vi "Data Array Length.vi"(10 "Read Tank Press":bool, 11 "Read Aux Flow":bool) -> (3 "Length":i32)   [LabVIEW 2019]
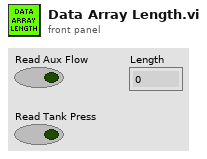
[diagram p1: front panel]
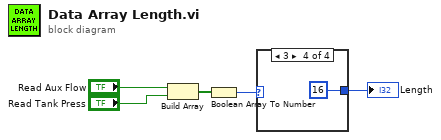
[diagram p0: block diagram]
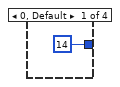
[diagram p2: hidden frame]
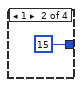
[diagram p3: hidden frame]
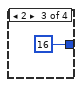
[diagram p4: hidden frame]
diagram:
  n1 = Build Array("Read Aux Flow", "Read Tank Press") -> (w1:bool[])
  n2 = Boolean Array To Number(Boolean array=w1) -> (number=w2:u32)
  n3 = case shown="3" w2 {
    tunnel: [14 ("length") 15 ("length") 16 ("length") 16 ("length")] -> w5
    frame 0, Default {
    }
    frame 1 {
    }
    frame 2 {
    }
    frame 3 {
    }
  }
  "Length" <- w5
